vi "JKISM++ Broadcast Status Change.vi"(0 "Status with Arguments":string, 5 "State(s) in (\"\")":string, 7 "Broadcast(T)":bool=TRUE) -> (6 "States Out":string)   [LabVIEW 2014, in "JKI-State-Machine-Plus.lvlib"]
doc: "Concatenates states in the JKI State Machine. Unwired inputs are safely ignored and will not be added to the state queue.\n\nFor instructions on how to use the JKI State Machine, examples and video tutorials, visit:\nhttp://jkisoft.com/state-machine/\n\n<B>Inputs:</B>\n <B>State(s) in Front:</B> This allows you to place new states in the front of the state machine queue. The default is an empty string.\n <B>State(s) in:</B> Wire the existing states to this input. The default is an empty string.\n <B>State(s) in Back:</B> This allows you to place new states in the back of the state machine queue. The default is an empty string.\n\n<B>Outputs:</B>\n <B>States Out:</B>This output returns a concatenation of all the inputs seperated by a line feed character. The line feed character is required by the JKI State Machine.\n\nJKI State Machine™ 2018.0.7.45\nhttp://jki.net/state-machine/\nCopyright (C) 2005-2018, JKI <info@jki.net>\nALL RIGHTS RESERVED"
uses:
  JKI-State-Machine-Plus.lvlib
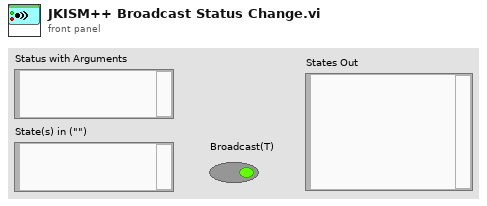
[diagram p1: front panel]
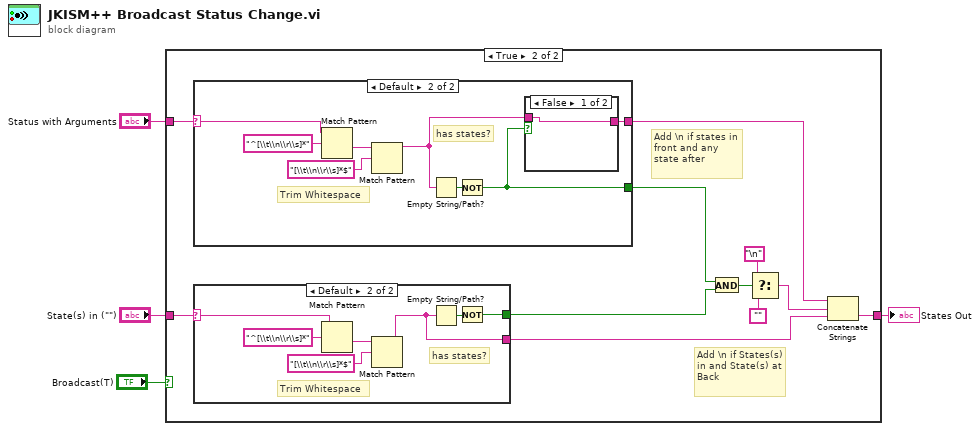
[diagram p0: block diagram]
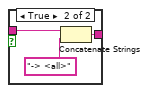
[diagram p5: hidden frame]
diagram:
  n1 = case shown="True" "Broadcast(T)" {
    tunnel: [w5 w16] -> w4
    tunnel: "Status with Arguments" -> [_ w8]
    tunnel: "State(s) in (\"\")" -> [w5 w7]
    frame False {
    }
    frame True {
      # "Add \\n if States(s) in and State(s) at Back"
      # "Add \\n if states in front and any state after"
      n2 = case shown="Default" w8 {
        selector: w8 -> [_ w27]
        tunnel: [_ w24] -> w15
        tunnel: [_ w25] -> w10
        frame "" {
        }
        frame Default {
          # "Trim Whitespace"
          # "has states?"
          n3 = Match Pattern(string=w27, regular expression="^[\\t\\n\\r\\s]*") -> (after substring=w29:string)  [unwired: 1 in, 3 out]
          n4 = Match Pattern(string=w29, regular expression="[\\t\\n\\r\\s]*$") -> (before substring=w26:string)  [unwired: 1 in, 3 out]
          n5 = Empty String/Path?(string/path=w26) -> (empty?=w31:bool)
          n6 = Not(x=w31) -> (.not. x?=w24:bool)
          n7 = case shown="False" w24 {
            tunnel: w26 -> [w32 w34]
            tunnel: [w32 w33] -> w25
            frame False {
            }
            frame True {
              n8 = Concatenate Strings(w34, "-> <all>" ("string")) -> (w33:string)
            }
          }
        }
      }
      n9 = case shown="Default" w7 {
        selector: w7 -> [_ w17]
        tunnel: [_ w22] -> w6
        tunnel: [_ w18] -> w9
        frame "" {
        }
        frame Default {
          # "Trim Whitespace"
          # "has states?"
          n10 = Match Pattern(string=w17, regular expression="^[\\t\\n\\r\\s]*") -> (after substring=w20:string)  [unwired: 1 in, 3 out]
          n11 = Match Pattern(string=w20, regular expression="[\\t\\n\\r\\s]*$") -> (before substring=w18:string)  [unwired: 1 in, 3 out]
          n12 = Empty String/Path?(string/path=w18) -> (empty?=w23:bool)
          n13 = Not(x=w23) -> (.not. x?=w22:bool)
        }
      }
      n14 = And(x=w15, y=w6) -> (x .and. y?=w14:bool)
      n15 = Select(t="\n", s=w14, f="") -> (s? t:f=w13:string)
      n16 = Concatenate Strings(w10, w13, w9) -> (w16:string)
    }
  }
  "States Out" <- w4
